vi "make_temp_files.vi"() -> ()   [LabVIEW 2012]
panel:
  in  "error in":errorcluster
  out "error out":errorcluster
  in  "Destination Path":path
  out "Number of Files found":i32
  in  "Source Path":path
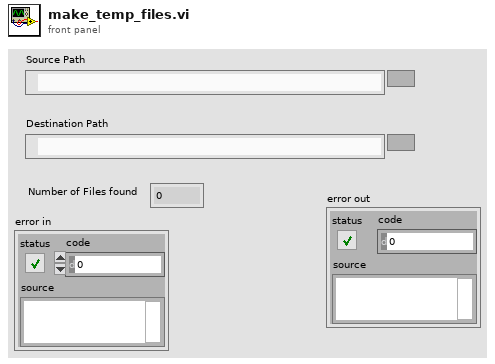
[diagram p1: front panel]
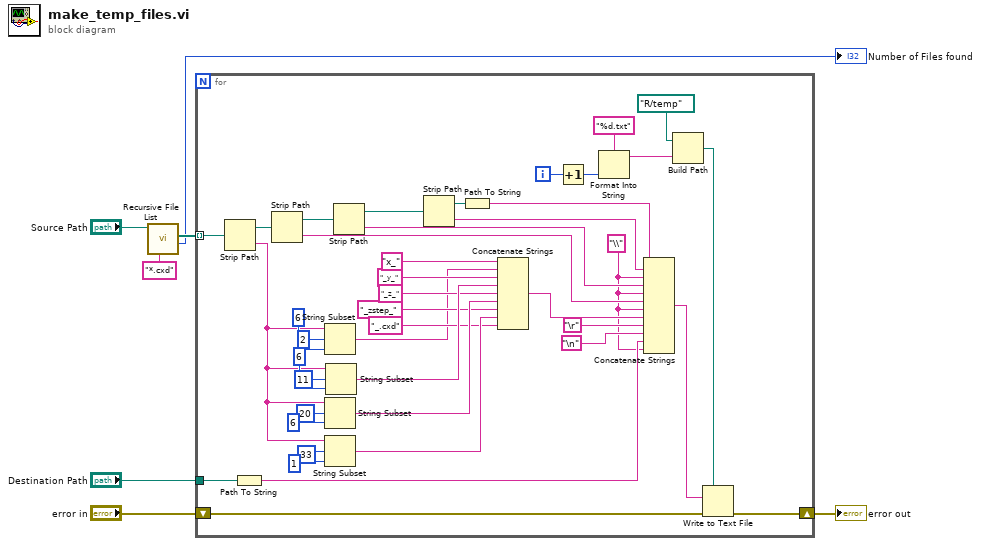
[diagram p0: block diagram]
diagram:
  n1 = call <vilib>:"Recursive File List.vi"("pattern"="*.cxd", "Folder Path"="Source Path") -> ("Number of Files"=→"Number of Files found":i32, "All Files in Dir"=w6:path[])  [unwired: 5 in, 3 out]
  n2 = for {
    tunnel: w6 -> [w23] mode=indexing
    tunnel: "Destination Path" -> [w17]
    shift-right: [w11] -> w1
    shift-left: "error in" -> [w12]
    i -> [w20]
    w8 = "\\" ("string")
    n3 = Strip Path(path=w23) -> (stripped path=w32:path, name=w37:string)
    n4 = Path To String(path=w17) -> (string=w16:string)
    n5 = Strip Path(path=w32) -> (stripped path=w31:path, name=w15:string)
    n6 = String Subset(string=w37, offset (0)=2, length (rest)=6 ("length (rest)")) -> (substring=w13:string)
    n7 = String Subset(string=w37, offset (0)=20, length (rest)=6 ("length (rest)")) -> (substring=w39:string)
    n8 = String Subset(string=w37, offset (0)=33, length (rest)=1 ("length (rest)")) -> (substring=w35:string)
    n9 = String Subset(string=w37, offset (0)=11, length (rest)=6 ("length (rest)")) -> (substring=w41:string)
    n10 = Strip Path(path=w31) -> (stripped path=w30:path, name=w28:string)
    n11 = Strip Path(path=w30) -> (stripped path=w10:path, name=w29:string)
    n12 = Path To String(path=w10) -> (string=w9:string)
    n13 = Concatenate Strings("x_" ("string"), w13, "_y_" ("string"), w41, "_z_" ("string"), w39, "_zstep_" ("string"), w35, "_.cxd" ("string")) -> (w14:string)
    n14 = Increment(x=w20) -> (x+1=w26:i32)
    n15 = Format Into String(format string="%d.txt", w26) -> (resulting string=w25:string)  [unwired: 2 in, 1 out]
    n16 = Concatenate Strings(w9, w29, w8, w28, w8, w15, w8, w14, "\r", "\n", w16, w8) -> (w21:string)
    n17 = Build Path(base path=path "R:/temp" ("file path (use dialog)"), name or relative path=w25) -> (appended path=w22:path)
    n18 = Write to Text File(file (use dialog)=w22, text=w21, error in=w12) -> (error out=w11:errorcluster)  [unwired: 1 in, 2 out]
  }
  "error out" <- w1
